vi "Modbus LDO Sensors.vi"(8 "error in":errorcluster, 11 "PLC Data":T1 {"PLC Data - LDO"."Timing"."Absolute Time" format="%<%H:%M:%S%3u>t"; "PLC Data - LDO"."Timing"."Display Time" format="%#.20f"; "PLC Data - LDO"."Timing"."Test Time Ref" format="%#.20f"; "PLC Data - LDO"."Timing"."Precondition Time Ref" format="%#.20f"; "PLC Data - LDO"."Timing"."First Call Time Ref" format="%#.20f"; "PLC Data - FVIR"."Timing"."Absolute Time" format="%<%H:%M:%S%3u>t"; "PLC Data - FVIR"."Timing"."Display Time" format="%#.20f"; "PLC Data - FVIR"."Timing"."Test Time Ref" format="%#.20f"; "PLC Data - FVIR"."Timing"."Precondition Time Ref" format="%#.20f"; "PLC Data - FVIR"."Timing"."First Call Time Ref" format="%#.20f"}) -> (0 "error out":errorcluster, 3 "PLC Data Output":T1 {"PLC Data - LDO"."Timing"."Absolute Time" format="%<%H:%M:%S%3u>t"; "PLC Data - LDO"."Timing"."Display Time" format="%#.20f"; "PLC Data - LDO"."Timing"."Test Time Ref" format="%#.20f"; "PLC Data - LDO"."Timing"."Precondition Time Ref" format="%#.20f"; "PLC Data - LDO"."Timing"."First Call Time Ref" format="%#.20f"; "PLC Data - FVIR"."Timing"."Absolute Time" format="%<%H:%M:%S%3u>t"; "PLC Data - FVIR"."Timing"."Display Time" format="%#.20f"; "PLC Data - FVIR"."Timing"."Test Time Ref" format="%#.20f"; "PLC Data - FVIR"."Timing"."Precondition Time Ref" format="%#.20f"; "PLC Data - FVIR"."Timing"."First Call Time Ref" format="%#.20f"})   [LabVIEW 2023, in "Modbus.lvlib"]
uses:
  Modbus.lvlib
  Modbus PLC Data All.ctl
  Modbus FVIR Control.ctl
  Modbus Timing.ctl
  <vilib>/Utility/miscctls.llb/LVDateTimeRec.ctl
  Modbus LDO Control.ctl
  WritingDataFile/Data to Save.ctl
  support/Terminate Conditions Cluster.ctl
panel:
  out "transposed array":string[][](array[string])
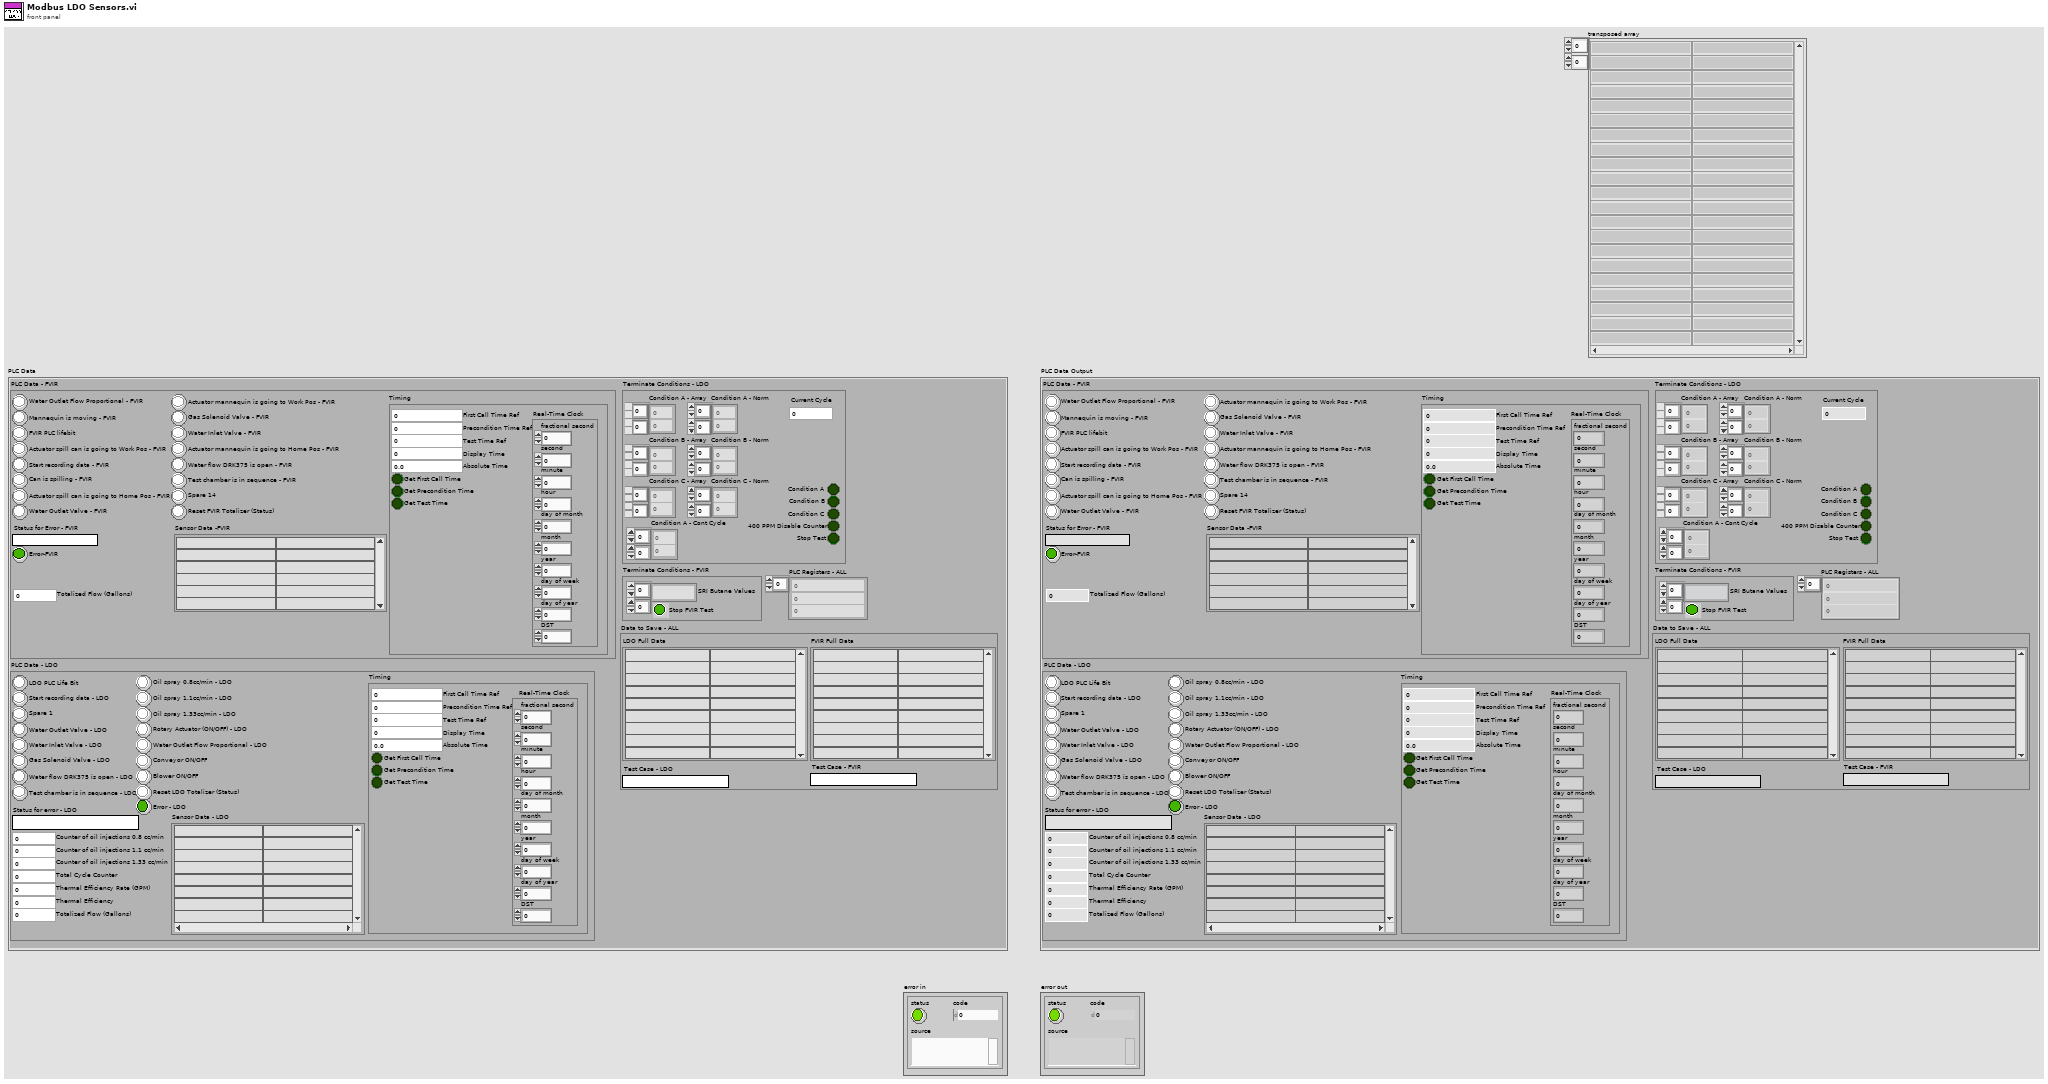
[diagram p1: front panel]
types:
  T1 = typedef "Modbus PLC Data All.ctl" = cluster{"PLC Data - FVIR":T2, "PLC Data - LDO":T5, "PLC Registers - ALL":i16[], "Data to Save - ALL":T6, "Terminate Conditions - LDO":T7, "Terminate Conditions - FVIR":cluster{"SRI Butane Values":string[][], "Stop FVIR Test":bool}}
  T2 = typedef "Modbus FVIR Control.ctl" = cluster{"Reset FVIR Totalizer (Status)":bool, "Spare 14":bool, "Actuator mannequin is going to Work Pos - FVIR":bool, "Actuator mannequin is going to Home Pos - FVIR":bool, "Test chamber is in sequence - FVIR ":bool, "Water flow DRK375 is open - FVIR":bool, "Gas Solenoid Valve - FVIR":bool, "Water Inlet Valve - FVIR":bool, "Water Outlet Flow Proportional - FVIR":bool, "Start recording data - FVIR":bool, "Actuator spill can is going to Work Pos - FVIR":bool, "Actuator spill can is going to Home Pos - FVIR":bool, "Water Outlet Valve - FVIR":bool, "Can is spilling - FVIR":bool, "Mannequin is moving - FVIR":bool, "FVIR PLC lifebit":bool, "Status for Error - FVIR":string, "Error-FVIR":bool, "Sensor Data -FVIR":string[][], "Totalized Flow (Gallons)":dbl, "Timing":T3}
  T3 = typedef "Modbus Timing.ctl" = cluster{"First Call Time Ref":dbl, "Precondition Time Ref":dbl, "Test Time Ref":dbl, "Get First Call Time":bool, "Get Precondition Time":bool, "Get Test Time":bool, "Display Time":dbl, "Real-Time Clock":T4, "Absolute Time":dbl}
  T4 = typedef "LVDateTimeRec.ctl" = cluster{"fractional second":dbl, "second":i32, "minute":i32, "hour":i32, "day of month":i32, "month":i32, "year":i32, "day of week":i32, "day of year":i32, "DST":i32}
  T5 = typedef "Modbus LDO Control.ctl" = cluster{"LDO PLC Life Bit":bool, "Start recording data - LDO":bool, "Spare 1":bool, "Water Outlet Valve - LDO":bool, "Water Inlet Valve - LDO":bool, "Gas Solenoid Valve - LDO":bool, "Water flow DRK375 is open - LDO":bool, "Test chamber is in sequence - LDO":bool, "Oil spray 0.8cc/min - LDO":bool, "Oil spray 1.1cc/min - LDO":bool, "Oil spray 1.33cc/min - LDO":bool, "Rotary Actuator (ON/OFF) - LDO":bool, "Water Outlet Flow Proportional - LDO":bool, "Conveyor ON/OFF":bool, "Blower ON/OFF":bool, "Reset LDO Totalizer (Status)":bool, "Status for error - LDO":string, "Error - LDO":bool, "Sensor Data - LDO":string[][], "Thermal Efficiency Rate (GPM)":dbl, "Thermal Efficiency":dbl, "Totalized Flow (Gallons)":dbl, "Counter of oil injections 1.33 cc/min":u16, "Total Cycle Counter":u16, "Counter of oil injections 1.1 cc/min":u16, "Counter of oil injections 0.8 cc/min":u16, "Timing":T3}
  T6 = typedef "Data to Save.ctl" = cluster{"LDO Full Data":string[][], "FVIR Full Data":string[][], "Test Case - FVIR":string, "Test Case - LDO":string}
  T7 = typedef "Terminate Conditions Cluster.ctl" = cluster{"Condition B - Array":dbl[][], "Current Cycle":u16, "Condition C - Array":dbl[][], "Condition A - Array":dbl[][], "400 PPM Disable Counter":bool, "Condition A - Norm":dbl[][], "Condition B - Norm":dbl[][], "Condition C - Norm":dbl[][], "Condition A":bool, "Condition B":bool, "Condition C":bool, "Condition A - Cont Cycle":dbl[][], "Stop Test":bool}
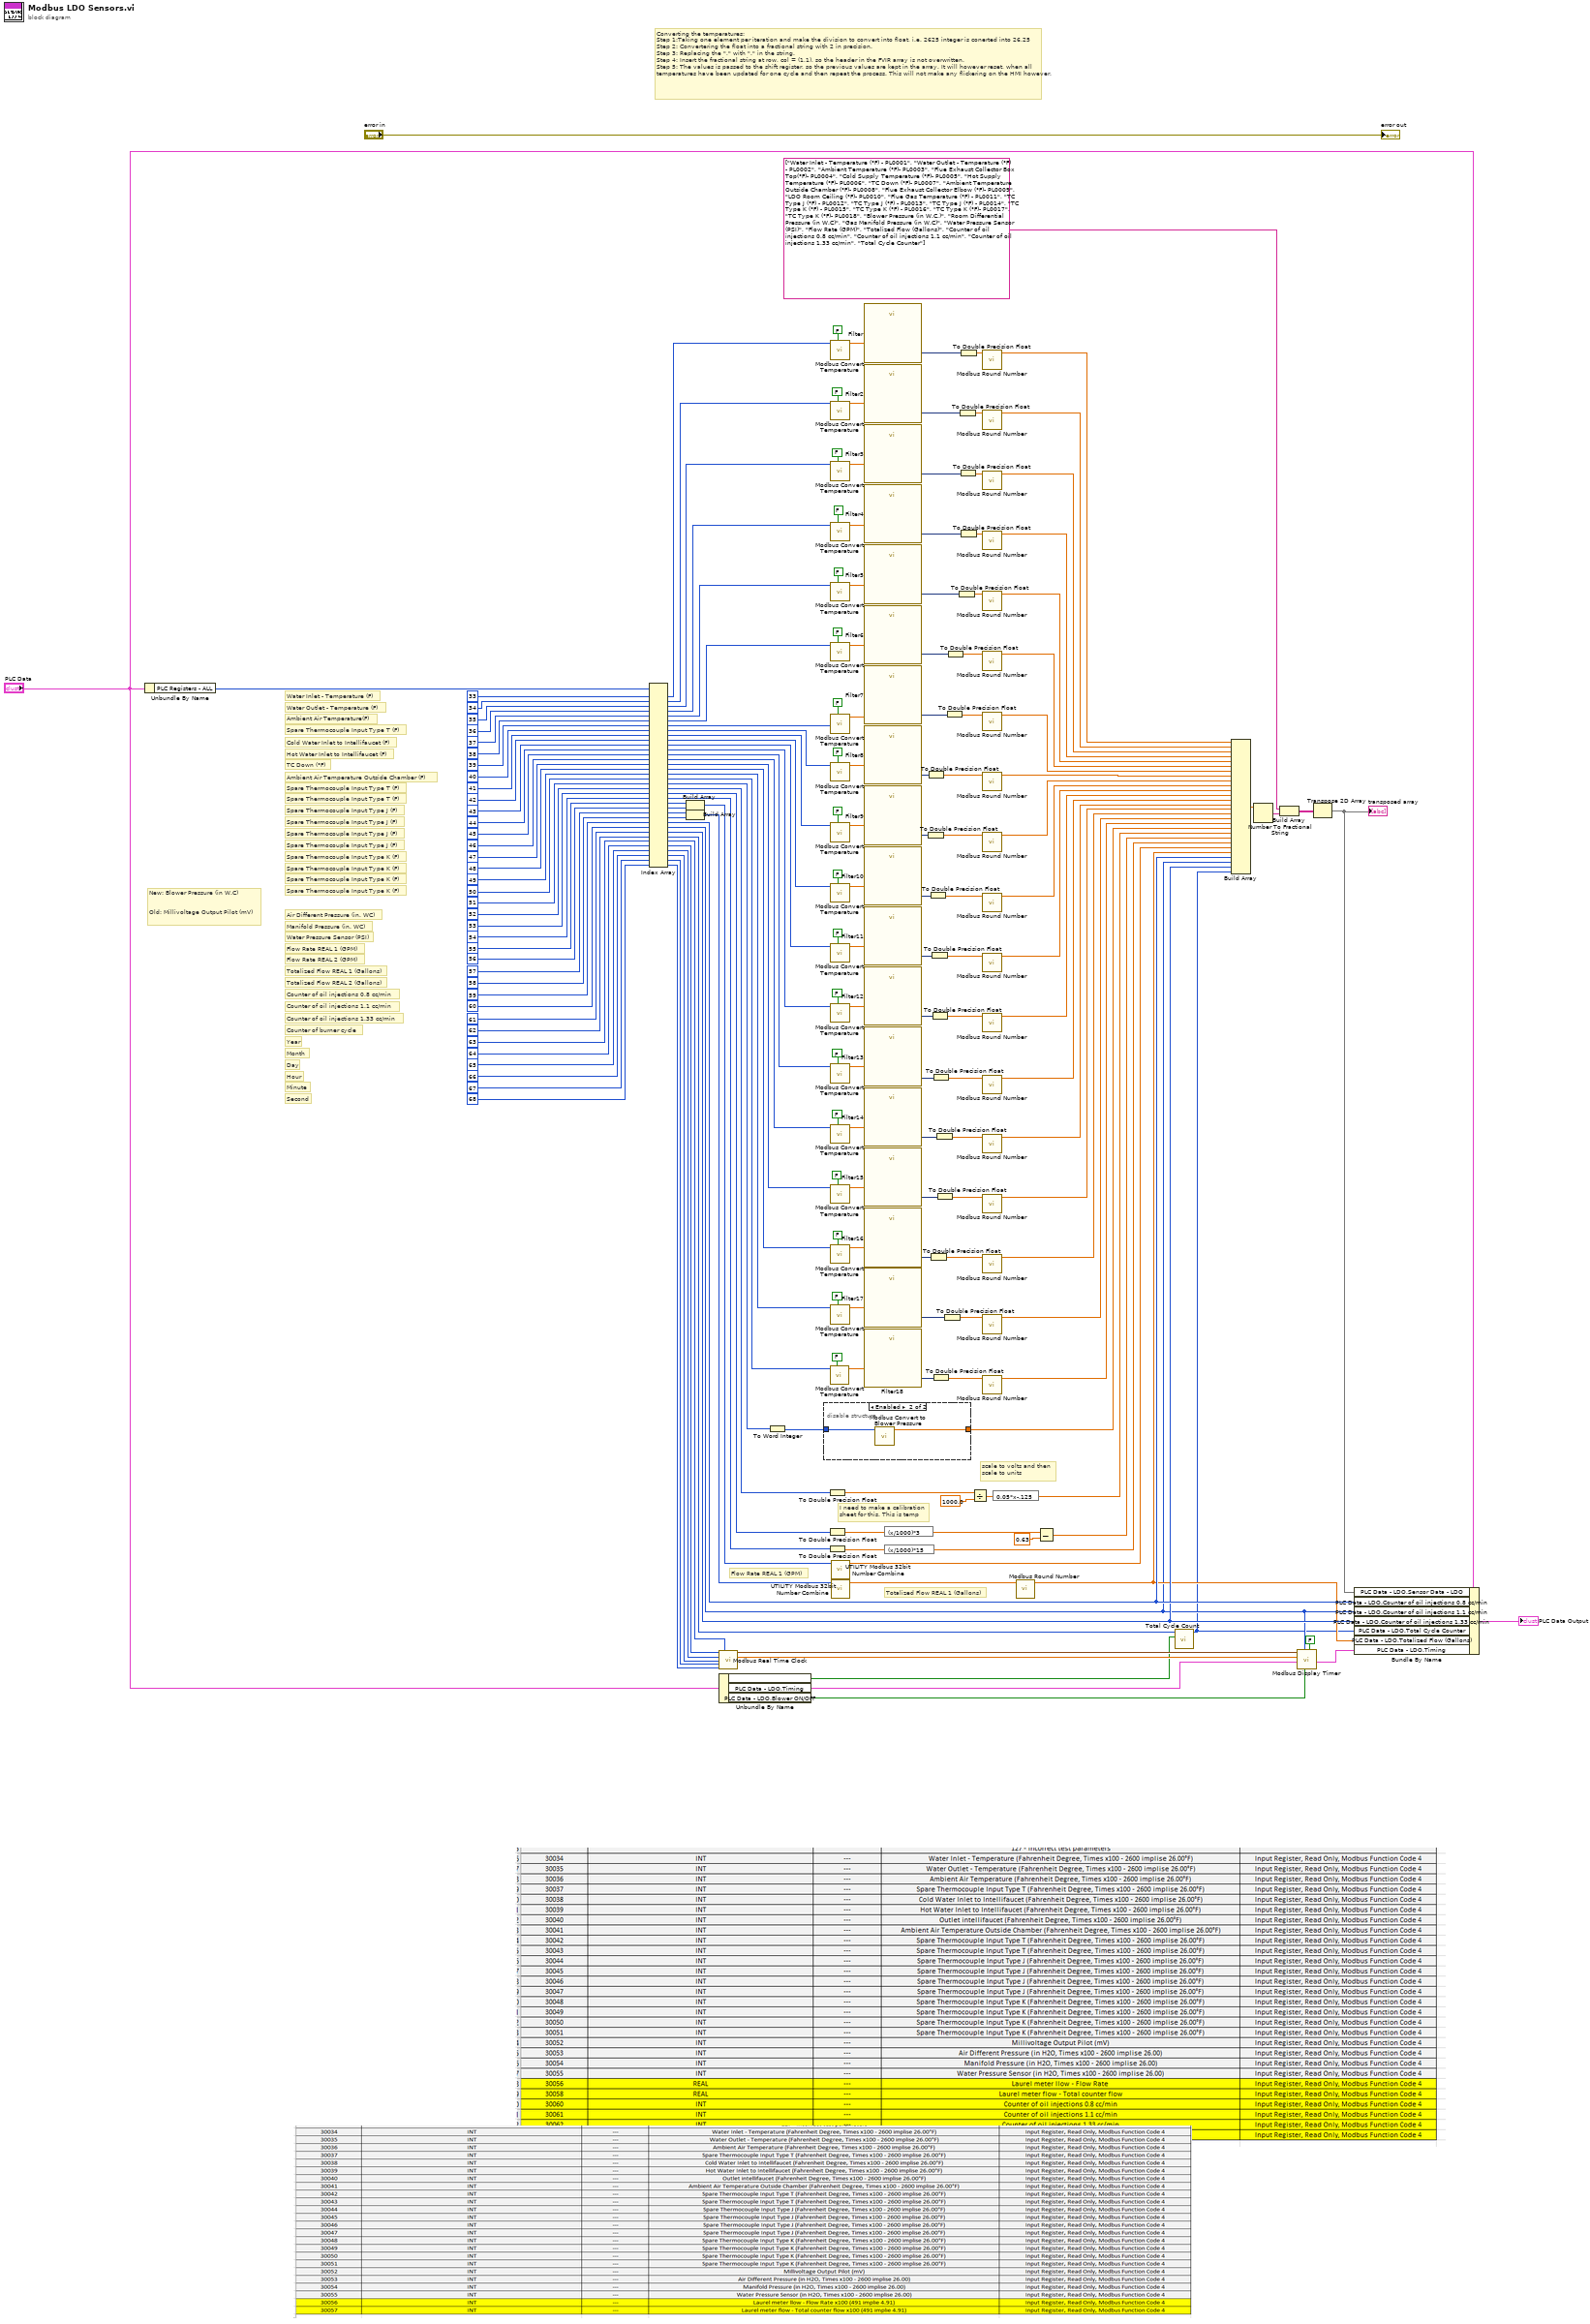
[diagram p0: block diagram]
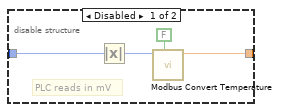
[diagram p2: hidden frame]
diagram:
  # "I need to make a calibration\nsheet for this. This is temp"
  # "Second"
  # "Minute"
  # "Hour"
  # "Day"
  # "Month"
  # "Year"
  # "Flow Rate REAL 1 (GPM)"
  # "Totalized Flow REAL 1 (Gallons)"
  # "Counter of burner cycle"
  # "Counter of oil injections 1.33 cc/min"
  # "Counter of oil injections 1.1 cc/min"
  # "Counter of oil injections 0.8 cc/min"
  # "Totalized Flow REAL 2 (Gallons)"
  # "Totalized Flow REAL 1 (Gallons)"
  # "scale to volts and then \nscale to units"
  # "Flow Rate REAL 2 (GPM)"
  # "Flow Rate REAL 1 (GPM)"
  # "Water Pressure Sensor (PSI)"
  # "Manifold Pressure (in. WC)"
  # "Air Different Pressure (in. WC)"
  # "New: Blower Pressure (in W.C)\n\n\nOld: Millivoltage Output Pilot (mV)"
  # "Spare Thermocouple Input Type K (F)"
  # "Spare Thermocouple Input Type K (F)"
  # "Spare Thermocouple Input Type K (F)"
  # "Spare Thermocouple Input Type K (F)"
  # "Spare Thermocouple Input Type J (F)"
  # "Spare Thermocouple Input Type J (F)"
  # "Spare Thermocouple Input Type J (F)"
  # "Spare Thermocouple Input Type J (F)"
  # "Spare Thermocouple Input Type T (F)"
  # "Spare Thermocouple Input Type T (F)"
  # "Ambient Air Temperature Outside Chamber (F)"
  # "TC Down (°F)"
  # "Hot Water Inlet to Intellifaucet (F)"
  # "Cold Water Inlet to Intellifaucet (F)"
  # "Spare Thermocouple Input Type T (F)"
  # "Ambient Air Temperature(F)"
  # "Water Outlet - Temperature (F)"
  # "Water Inlet - Temperature (F)"
  # "Converting the temperatures: \nStep 1:Taking one element per iteration and make the division to convert into float, i.e. 2625 integer is conerted into 26,25\nStep 2: Convertering the float into a fractional string with 2 in precision. \nStep 3: Replacing the \",\" with \".\" in the string.\nStep 4: Insert the fractional string at row, col = (1,1), so the header in the FVIR array is not overwritten. \nStep 5: The values is passed to the shift register, so the previous values are kept in the array. It will however reset, when all temperatures have been updated for one cycle and then repeat the process. This will not make any flickering on the HMI however."
  n1 = Unbundle By Name("PLC Data") -> ("PLC Registers - ALL"=w145:i16[])
  n2 = Index Array(array=w145, index #1=33 ("index"), index #2=34 ("index"), index #3=35 ("index"), index #4=36 ("index"), index #5=37 ("index"), index #6=38 ("index"), index #7=39 ("index"), index #8=40 ("index"), index #9=41 ("index"), index #10=42 ("index"), index #11=43 ("index"), index #12=44 ("index"), index #13=45 ("index"), index #14=46 ("index"), index #15=47 ("index"), index #16=48 ("index"), index #17=49 ("index"), index #18=50 ("index"), index #19=51 ("index"), index #20=52 ("index"), index #21=53 ("index"), index #22=54 ("index"), index #23=55 ("index"), index #24=56 ("index"), index #25=57 ("index"), index #26=58 ("index"), index #27=59 ("index"), index #28=60 ("index"), index #29=61 ("index"), index #30=62 ("index"), index #31=63 ("index"), index #32=64 ("index"), index #33=65 ("index"), index #34=66 ("index"), index #35=67 ("index"), index #36=68 ("index")) -> (element #1=w172:i16, element #2=w171:i16, element #3=w170:i16, element #4=w169:i16, element #5=w168:i16, element #6=w167:i16, element #7=w166:i16, element #8=w165:i16, element #9=w164:i16, element #10=w163:i16, element #11=w162:i16, element #12=w161:i16, element #13=w160:i16, element #14=w159:i16, element #15=w158:i16, element #16=w157:i16, element #17=w156:i16, element #18=w155:i16, element #19=w68:i16, element #20=w153:i16, element #21=w144:i16, element #22=w152:i16, element #23=w42:i16, element #24=w41:i16, element #25=w40:i16, element #26=w39:i16, element #27=w35:i16, element #28=w20:i16, element #29=w34:i16, element #30=w33:i16, element #31=w24:i16, element #32=w23:i16, element #33=w22:i16, element #34=w13:i16, element #35=w12:i16, element #36=w11:i16)
  n3 = Build Array(w42, w41) -> (w38:i16[])
  n4 = Build Array(w40, w39) -> (w37:i16[])
  n5 = call "Modbus Real Time Clock.vi"("Month"=w23, "Year"=w24, "Day"=w22, "Hour"=w13, "Minute"=w12, "Second"=w11) -> ("Real-Time Clock"=w8:T4, "Absolute Time"=w9:dbl)  [unwired: 8 in]
  n6 = Unbundle By Name("PLC Data") -> ("PLC Data - LDO.Water Outlet Valve - LDO"=w7:bool, "PLC Data - LDO.Timing"=w10:T3, "PLC Data - LDO.Blower ON/OFF"=w21:bool)
  n7 = To Word Integer(number=w68) -> (16bit integer=w14:i16)
  n8 = disable-structure shown="Enabled" {
    disable-tunnel: [w199 w201] -> w49
    disable-tunnel: w14 -> [w198 w202]
    frame Disabled {
      # "PLC reads in mV"
      n9 = Absolute Value(x=w198) -> (abs(x)=w197:i16)
      n10 = call "Modbus Convert Temperature.vi"("Divide by 100?"=FALSE, "PLC Value"=w197) -> ("Converted Value"=w199:dbl)  [unwired: 8 in, 1 out]
    }
    frame Enabled {
      n11 = call "Modbus Convert to Blower Pressure.vi"("Blower Voltage Output (mV)"=w202) -> ("Blower Pressure (in. W.C)"=w201:dbl)  [unwired: 10 in]
    }
  }
  n12 = To Double Precision Float(number=w153) -> (double precision float=w17:dbl)
  n13 = To Double Precision Float(number=w144) -> (double precision float=w143:dbl)
  n14 = To Double Precision Float(number=w152) -> (double precision float=w4:dbl)
  n15 = call "Modbus Convert Temperature.vi"("Divide by 100?"=FALSE, "PLC Value"=w155) -> ("Converted Value"=w105:dbl)  [unwired: 8 in, 1 out]
  n16 = call "Modbus Convert Temperature.vi"("Divide by 100?"=FALSE, "PLC Value"=w172) -> ("Converted Value"=w140:dbl)  [unwired: 8 in, 1 out]
  n17 = call "Modbus Convert Temperature.vi"("Divide by 100?"=FALSE, "PLC Value"=w171) -> ("Converted Value"=w137:dbl)  [unwired: 8 in, 1 out]
  n18 = call "Modbus Convert Temperature.vi"("Divide by 100?"=FALSE, "PLC Value"=w170) -> ("Converted Value"=w135:dbl)  [unwired: 8 in, 1 out]
  n19 = call "Modbus Convert Temperature.vi"("Divide by 100?"=FALSE, "PLC Value"=w169) -> ("Converted Value"=w133:dbl)  [unwired: 8 in, 1 out]
  n20 = call "Modbus Convert Temperature.vi"("Divide by 100?"=FALSE, "PLC Value"=w168) -> ("Converted Value"=w131:dbl)  [unwired: 8 in, 1 out]
  n21 = call "Modbus Convert Temperature.vi"("Divide by 100?"=FALSE, "PLC Value"=w167) -> ("Converted Value"=w129:dbl)  [unwired: 8 in, 1 out]
  n22 = call "Modbus Convert Temperature.vi"("Divide by 100?"=FALSE, "PLC Value"=w166) -> ("Converted Value"=w127:dbl)  [unwired: 8 in, 1 out]
  n23 = call "Modbus Convert Temperature.vi"("Divide by 100?"=FALSE, "PLC Value"=w165) -> ("Converted Value"=w125:dbl)  [unwired: 8 in, 1 out]
  n24 = call "Modbus Convert Temperature.vi"("Divide by 100?"=FALSE, "PLC Value"=w164) -> ("Converted Value"=w123:dbl)  [unwired: 8 in, 1 out]
  n25 = call "Modbus Convert Temperature.vi"("Divide by 100?"=FALSE, "PLC Value"=w163) -> ("Converted Value"=w121:dbl)  [unwired: 8 in, 1 out]
  n26 = call "Modbus Convert Temperature.vi"("Divide by 100?"=FALSE, "PLC Value"=w162) -> ("Converted Value"=w119:dbl)  [unwired: 8 in, 1 out]
  n27 = call "Modbus Convert Temperature.vi"("Divide by 100?"=FALSE, "PLC Value"=w161) -> ("Converted Value"=w117:dbl)  [unwired: 8 in, 1 out]
  n28 = call "Modbus Convert Temperature.vi"("Divide by 100?"=FALSE, "PLC Value"=w160) -> ("Converted Value"=w115:dbl)  [unwired: 8 in, 1 out]
  n29 = call "Modbus Convert Temperature.vi"("Divide by 100?"=FALSE, "PLC Value"=w159) -> ("Converted Value"=w113:dbl)  [unwired: 8 in, 1 out]
  n30 = call "Modbus Convert Temperature.vi"("Divide by 100?"=FALSE, "PLC Value"=w158) -> ("Converted Value"=w111:dbl)  [unwired: 8 in, 1 out]
  n31 = call "Modbus Convert Temperature.vi"("Divide by 100?"=FALSE, "PLC Value"=w157) -> ("Converted Value"=w109:dbl)  [unwired: 8 in, 1 out]
  n32 = call "Modbus Convert Temperature.vi"("Divide by 100?"=FALSE, "PLC Value"=w156) -> ("Converted Value"=w107:dbl)  [unwired: 8 in, 1 out]
  n33 = call "UTILITY Modbus 32bit Number Combine.vi"("Holding Registers"=w38) -> ("Data"=w36:sgl)  [unwired: 9 in, 1 out]
  n34 = call "UTILITY Modbus 32bit Number Combine.vi"("Holding Registers"=w37) -> ("Data"=w31:sgl)  [unwired: 9 in, 1 out]
  n35 = call "Filter"("Signal"=w140) -> ("Filtered Signal"=w139:dynamicdata)  [unwired: 9 in, 1 out]
  n36 = call "Filter2"("Signal"=w137) -> ("Filtered Signal"=w138:dynamicdata)  [unwired: 9 in, 1 out]
  n37 = call "Filter3"("Signal"=w135) -> ("Filtered Signal"=w136:dynamicdata)  [unwired: 9 in, 1 out]
  n38 = call "Filter4"("Signal"=w133) -> ("Filtered Signal"=w134:dynamicdata)  [unwired: 9 in, 1 out]
  n39 = call "Filter5"("Signal"=w131) -> ("Filtered Signal"=w132:dynamicdata)  [unwired: 9 in, 1 out]
  n40 = call "Filter6"("Signal"=w129) -> ("Filtered Signal"=w130:dynamicdata)  [unwired: 9 in, 1 out]
  n41 = call "Filter7"("Signal"=w127) -> ("Filtered Signal"=w128:dynamicdata)  [unwired: 9 in, 1 out]
  n42 = call "Filter8"("Signal"=w125) -> ("Filtered Signal"=w126:dynamicdata)  [unwired: 9 in, 1 out]
  n43 = call "Filter9"("Signal"=w123) -> ("Filtered Signal"=w124:dynamicdata)  [unwired: 9 in, 1 out]
  n44 = call "Filter10"("Signal"=w121) -> ("Filtered Signal"=w122:dynamicdata)  [unwired: 9 in, 1 out]
  n45 = call "Filter11"("Signal"=w119) -> ("Filtered Signal"=w120:dynamicdata)  [unwired: 9 in, 1 out]
  n46 = call "Filter12"("Signal"=w117) -> ("Filtered Signal"=w118:dynamicdata)  [unwired: 9 in, 1 out]
  n47 = call "Filter13"("Signal"=w115) -> ("Filtered Signal"=w116:dynamicdata)  [unwired: 9 in, 1 out]
  n48 = call "Filter14"("Signal"=w113) -> ("Filtered Signal"=w114:dynamicdata)  [unwired: 9 in, 1 out]
  n49 = call "Filter15"("Signal"=w111) -> ("Filtered Signal"=w112:dynamicdata)  [unwired: 9 in, 1 out]
  n50 = call "Filter16"("Signal"=w109) -> ("Filtered Signal"=w110:dynamicdata)  [unwired: 9 in, 1 out]
  n51 = call "Filter17"("Signal"=w107) -> ("Filtered Signal"=w108:dynamicdata)  [unwired: 9 in, 1 out]
  n52 = call "Filter18"("Signal"=w105) -> ("Filtered Signal"=w106:dynamicdata)  [unwired: 9 in, 1 out]
  n53 = expression code="(x/1000)*3"(w143) -> (w3:dbl)
  n54 = expression code="(x/1000)*15"(w4) -> (w141:dbl)
  n55 = To Double Precision Float(number=w124) -> (double precision float=w88:dbl)
  n56 = To Double Precision Float(number=w126) -> (double precision float=w90:dbl)
  n57 = To Double Precision Float(number=w122) -> (double precision float=w86:dbl)
  n58 = To Double Precision Float(number=w110) -> (double precision float=w74:dbl)
  n59 = To Double Precision Float(number=w120) -> (double precision float=w84:dbl)
  n60 = To Double Precision Float(number=w118) -> (double precision float=w82:dbl)
  n61 = To Double Precision Float(number=w116) -> (double precision float=w80:dbl)
  n62 = To Double Precision Float(number=w106) -> (double precision float=w70:dbl)
  n63 = To Double Precision Float(number=w114) -> (double precision float=w78:dbl)
  n64 = To Double Precision Float(number=w112) -> (double precision float=w76:dbl)
  n65 = To Double Precision Float(number=w108) -> (double precision float=w72:dbl)
  n66 = To Double Precision Float(number=w128) -> (double precision float=w92:dbl)
  n67 = To Double Precision Float(number=w130) -> (double precision float=w94:dbl)
  n68 = To Double Precision Float(number=w132) -> (double precision float=w96:dbl)
  n69 = To Double Precision Float(number=w138) -> (double precision float=w102:dbl)
  n70 = To Double Precision Float(number=w136) -> (double precision float=w100:dbl)
  n71 = To Double Precision Float(number=w139) -> (double precision float=w104:dbl)
  n72 = To Double Precision Float(number=w134) -> (double precision float=w98:dbl)
  n73 = Divide(x=w17, y=1000.0) -> (x/y=w15:dbl)
  n74 = call "Modbus Round Number.vi"("Number"=w104) -> ("Rounded Number"=w103:dbl)  [unwired: 10 in]
  n75 = call "Modbus Round Number.vi"("Number"=w102) -> ("Rounded Number"=w101:dbl)  [unwired: 10 in]
  n76 = call "Modbus Round Number.vi"("Number"=w100) -> ("Rounded Number"=w99:dbl)  [unwired: 10 in]
  n77 = call "Modbus Round Number.vi"("Number"=w98) -> ("Rounded Number"=w97:dbl)  [unwired: 10 in]
  n78 = call "Modbus Round Number.vi"("Number"=w96) -> ("Rounded Number"=w95:dbl)  [unwired: 10 in]
  n79 = call "Modbus Round Number.vi"("Number"=w94) -> ("Rounded Number"=w93:dbl)  [unwired: 10 in]
  n80 = call "Modbus Round Number.vi"("Number"=w92) -> ("Rounded Number"=w91:dbl)  [unwired: 10 in]
  n81 = call "Modbus Round Number.vi"("Number"=w90) -> ("Rounded Number"=w89:dbl)  [unwired: 10 in]
  n82 = call "Modbus Round Number.vi"("Number"=w88) -> ("Rounded Number"=w87:dbl)  [unwired: 10 in]
  n83 = call "Modbus Round Number.vi"("Number"=w86) -> ("Rounded Number"=w85:dbl)  [unwired: 10 in]
  n84 = call "Modbus Round Number.vi"("Number"=w84) -> ("Rounded Number"=w83:dbl)  [unwired: 10 in]
  n85 = call "Modbus Round Number.vi"("Number"=w82) -> ("Rounded Number"=w81:dbl)  [unwired: 10 in]
  n86 = call "Modbus Round Number.vi"("Number"=w80) -> ("Rounded Number"=w79:dbl)  [unwired: 10 in]
  n87 = call "Modbus Round Number.vi"("Number"=w78) -> ("Rounded Number"=w77:dbl)  [unwired: 10 in]
  n88 = call "Modbus Round Number.vi"("Number"=w76) -> ("Rounded Number"=w75:dbl)  [unwired: 10 in]
  n89 = call "Modbus Round Number.vi"("Number"=w74) -> ("Rounded Number"=w73:dbl)  [unwired: 10 in]
  n90 = call "Modbus Round Number.vi"("Number"=w72) -> ("Rounded Number"=w71:dbl)  [unwired: 10 in]
  n91 = call "Modbus Round Number.vi"("Number"=w70) -> ("Rounded Number"=w69:dbl)  [unwired: 10 in]
  n92 = expression code="0.05*x-.125"(w15) -> (w142:dbl)
  n93 = call "Modbus Round Number.vi"("Number"=w31) -> ("Rounded Number"=w32:dbl)  [unwired: 10 in]
  n94 = Subtract(x=w3, y=0.63) -> (x-y=w1:dbl)
  n95 = call "Total Cycle Count.vi"("Water Outlet Valve - LDO"=w7, "Counter of burner cycle"=w33) -> ("Total Cycle Count"=w19:u16)  [unwired: 9 in]
  n96 = Build Array(w103, w101, w99, w97, w95, w93, w91, w89, w87, w85, w83, w81, w79, w77, w75, w73, w71, w69, w49, w142, w1, w141, w36, w32, w35, w20, w34, w19) -> (w151:dbl[])
  n97 = Number To Fractional String(number=w151) -> (F-format string=w150:string[])  [unwired: 3 in]
  n98 = Build Array(string[] ["Water Inlet - Temperature (°F) - PL0001", "Water Outlet - Temperature (°F) - PL0002", "Ambient Temperature (°F)- PL0003", "Flue Exhaust Collector Box Top(°F)- PL0004", "Cold Supply Temperature (°F)- PL0005", "Hot Supply Temperature (°F)- PL0006", "TC Down (°F)- PL0007", "Ambient Temperature Outside Chamber (°F)- PL0008", "Flue Exhaust Collector Elbow (°F)- PL0009", "LDO Room Ceiling (°F)- PL0010", "Flue Gas Temperature (°F) - PL0011", "TC Type J (°F) - PL0012", "TC Type J (°F) - PL0013", "TC Type J (°F) - PL0014", "TC Type K (°F) - PL0015", "TC Type K (°F) - PL0016", "TC Type K (°F)- PL0017", "TC Type K (°F)- PL0018", "Blower Pressure (in W.C.)", "Room Differential Pressure (in W.C)", "Gas Manifold Pressure (in W.C)", "Water Pressure Sensor (PSI)", "Flow Rate (GPM)", "Totalized Flow (Gallons)", "Counter of oil injections 0.8 cc/min", "Counter of oil injections 1.1 cc/min", "Counter of oil injections 1.33 cc/min", "Total Cycle Counter"] ("Array 2"), w150) -> (w148:string[][])
  n99 = call "Modbus Display Timer.vi"("FVIR?"=FALSE, "Blower ON/OFF"=w21, "Counter of oil injections 1.1 cc/min"=w20, "Timing in"=w10, "Absolute Time"=w9, "Real-Time Clock"=w8) -> ("Timing Out"=w5:T3)  [unwired: 5 in]
  n100 = Transpose 2D Array(2D array=w148) -> (transposed array=w147:string[][])
  "transposed array" <- w147
  n101 = Bundle By Name(cluster="PLC Data", "PLC Data - LDO.Sensor Data - LDO"=w147, "PLC Data - LDO.Counter of oil injections 0.8 cc/min"=w35, "PLC Data - LDO.Counter of oil injections 1.1 cc/min"=w20, "PLC Data - LDO.Counter of oil injections 1.33 cc/min"=w34, "PLC Data - LDO.Total Cycle Counter"=w19, "PLC Data - LDO.Totalized Flow (Gallons)"=w32, "PLC Data - LDO.Timing"=w5) -> (→"PLC Data Output":T1)
  "error out" <- "error in"
